vi "FileIO-Parameter Folder.vi"(3 "create if doesn't exist (T)":bool=TRUE, 4 "subfolder":string="EPL\\SUV\\Level Sweep") -> (1 "parameter folder":path)   [LabVIEW 2020]
uses:
  <vilib>/Utility/sysdir.llb/System Directory Type.ctl
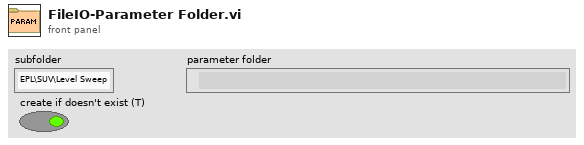
[diagram p1: front panel]
types:
  T1 = typedef "System Directory Type.ctl" = i32
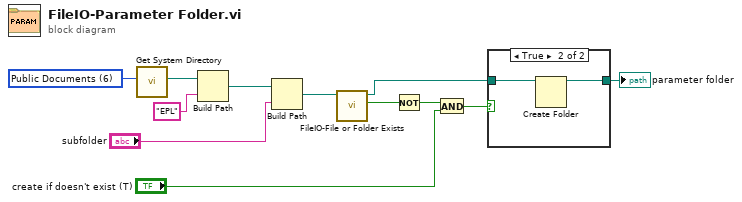
[diagram p0: block diagram]
diagram:
  w12 = T1 6 items=["User Home", "User Desktop", "User Documents", "User Application Data", "User Preferences", "User Temporary", "Public Documents", "Public Application Data", "Public Preferences", "System Core Libraries", "System Installed Libraries", "Application Files", "Boot Volume Root"] ("system directory type")
  n1 = call <vilib>:"Get System Directory.vi"("system directory type"=w12) -> ("system directory"=w11:path)  [unwired: 10 in]
  n2 = Build Path(base path=w11, name or relative path="EPL") -> (appended path=w9:path)
  n3 = Build Path(base path=w9, name or relative path="subfolder") -> (appended path=w7:path)
  n4 = call "FileIO-File or Folder Exists.vi"("path"=w7) -> ("Directory?"=w6:bool, "dup path"=w2:path)  [unwired: 7 in, 2 out]
  n5 = Not(x=w6) -> (.not. x?=w5:bool)
  n6 = And(x=w5, y="create if doesn't exist (T)") -> (x .and. y?=w3:bool)
  n7 = case shown="True" w3 {
    tunnel: w2 -> [w13 w15]
    tunnel: [w13 w14] -> w1
    frame False {
    }
    frame True {
      n8 = Create Folder(path (use dialog)=w15) -> (created path=w14:path)  [unwired: 2 in, 2 out]
    }
  }
  "parameter folder" <- w1
